vi "Main.vi"() -> ()   [LabVIEW 2020]
doc: "Application created to graph orbital movement of Venus, Earth, Mars and show distances and time needed for information to flow between them."
uses:
  Type Definitions/StateMachineEnum.ctl
  Variables/Stop-bool.vi
  Variables/Phi-initial.vi
panel:
  in  "Hiding button 2":bool
  in  "Hiding button":bool
  out "t S-E":string
  out "t M-E":string
  out "t S-M":string
  out "t V-M":string
  out "t S-V":string
  out "t V-E":string
  out "d M-E":dbl format="%.3g"
  out "d V-E":dbl format="%#.3g"
  out "d V-M":dbl format="%#.3g"
  out "d S-E":dbl format="%.3g"
  out "d S-M":dbl format="%.3g"
  out "d S-V":dbl format="%.3g"
  in  "Pause":bool
  out "Fi earth":dbl format="%#.4g"
  out "R earth":dbl format="%.4g"
  out "Fi mars":dbl format="%#.4g"
  out "R mars":dbl format="%.4g"
  out "Fi venus":dbl format="%#.4g"
  out "R venus":dbl format="%.4g"
  in  "Save Data":bool
  in  "Graphing speed":dbl(slide) scale=1.0..100.0
  out "XY Graph":cluster{dbl[], dbl[]}[](graph)
  in  "Stop drawing":bool
  in  "Draw Graph":bool
  in  "Exit":bool
  in  "Settings":bool
  # "Positions of planets"
  # "R [AU]"
  # "fi [deg]"
  # "Venus"
  # "Mars"
  # "Earth"
  # "Distances in AU (upper triangle) and time min::s::ms (lower triangle)"
  # "Sun"
  # "Venus"
  # "Mars"
  # "Earth"
  # "Sun"
  # "Venus"
  # "Mars"
  # "Earth"
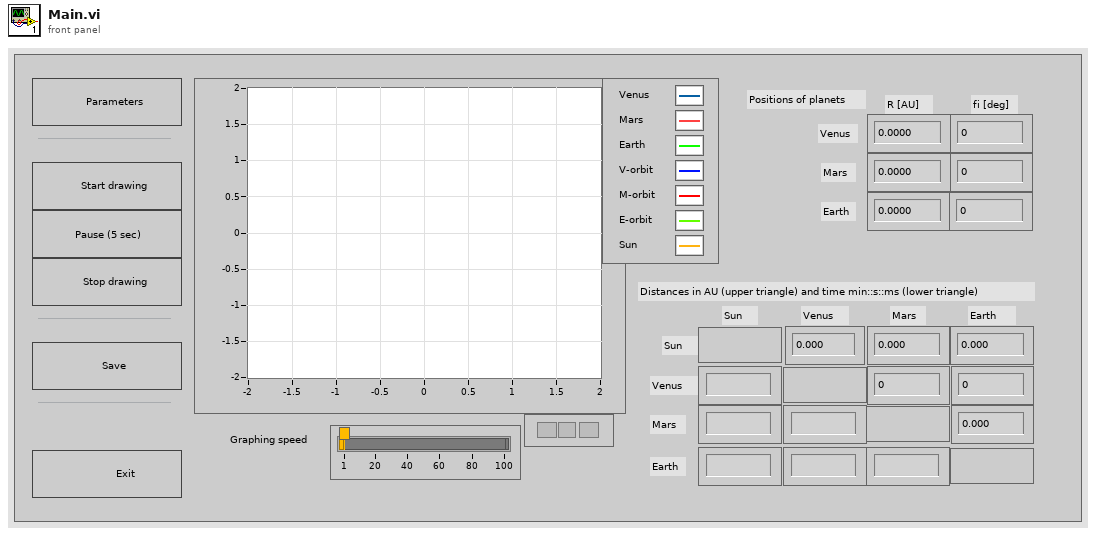
[diagram p1: front panel]
types:
  T1 = typedef "StateMachineEnum.ctl" = enum16{"Initialize", "Wait for event", "Draw graph", "Exit", "Save Data"}
  T2 = cluster{"t V-E":string, "t S-V":string, "t V-M":string, "t S-M":string, "t M-E":string, "t S-E":string}
  T3 = cluster{"d V-E":dbl, "d S-V":dbl, "d V-M":dbl, "d S-M":dbl, "d M-E":dbl, "d S-E":dbl}
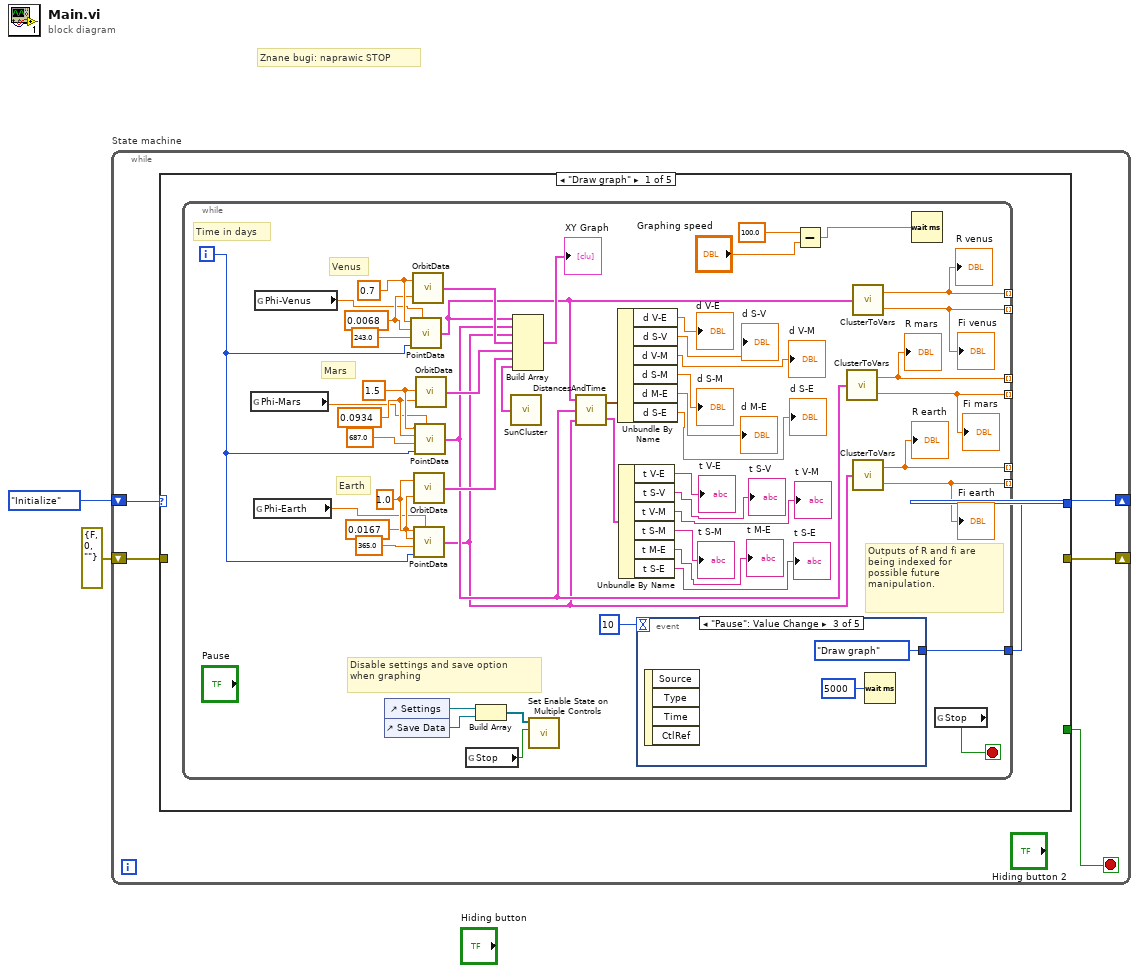
[diagram p0: block diagram]
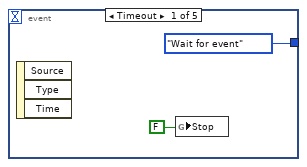
[diagram p2: hidden frame]
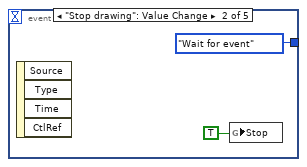
[diagram p3: hidden frame]
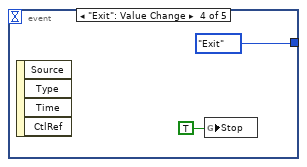
[diagram p4: hidden frame]
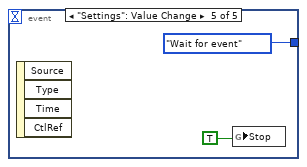
[diagram p5: hidden frame]
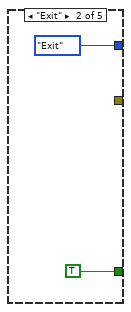
[diagram p6: hidden frame]
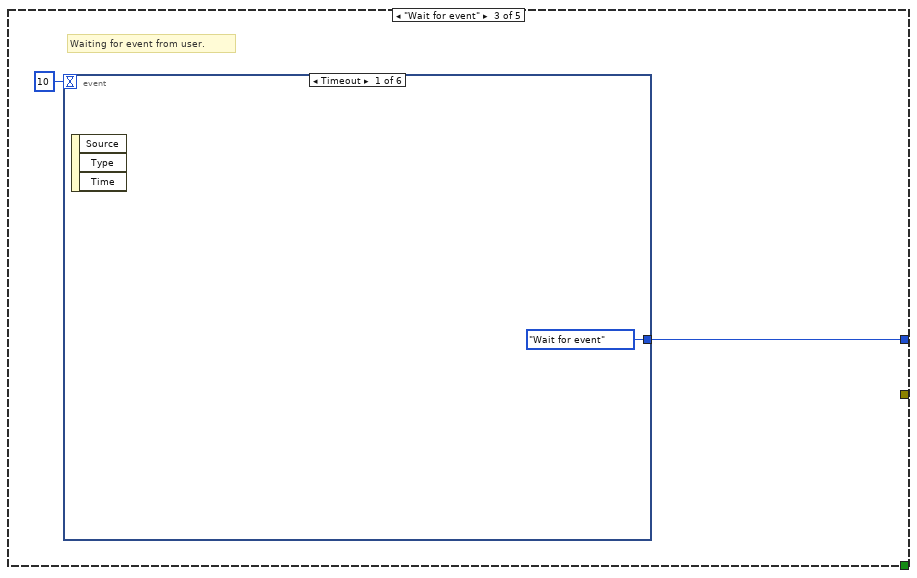
[diagram p7: hidden frame]
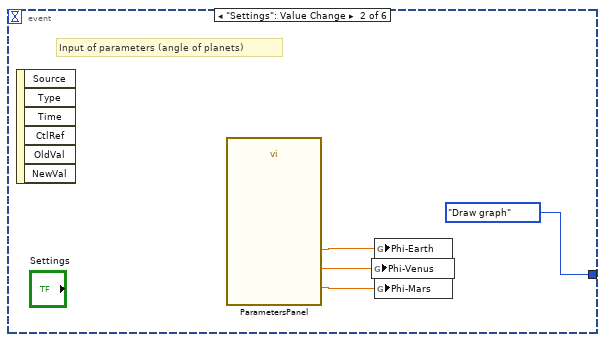
[diagram p8: hidden frame]
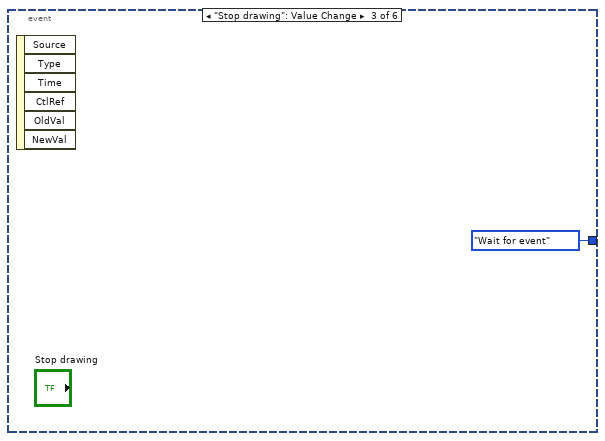
[diagram p9: hidden frame]
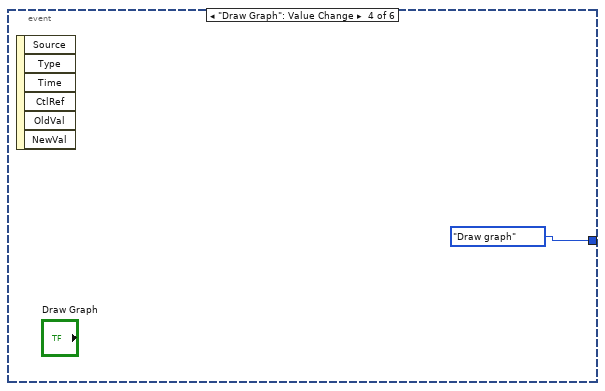
[diagram p10: hidden frame]
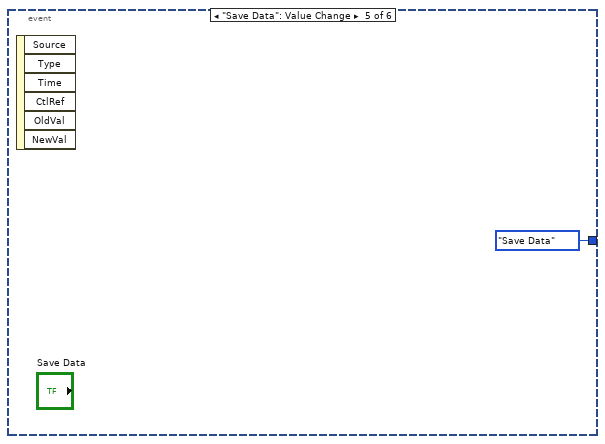
[diagram p11: hidden frame]
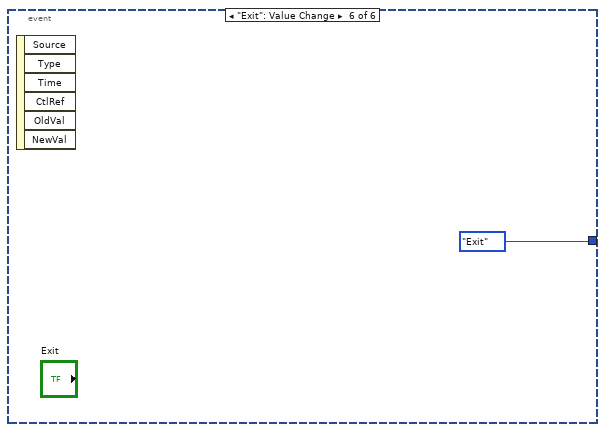
[diagram p12: hidden frame]
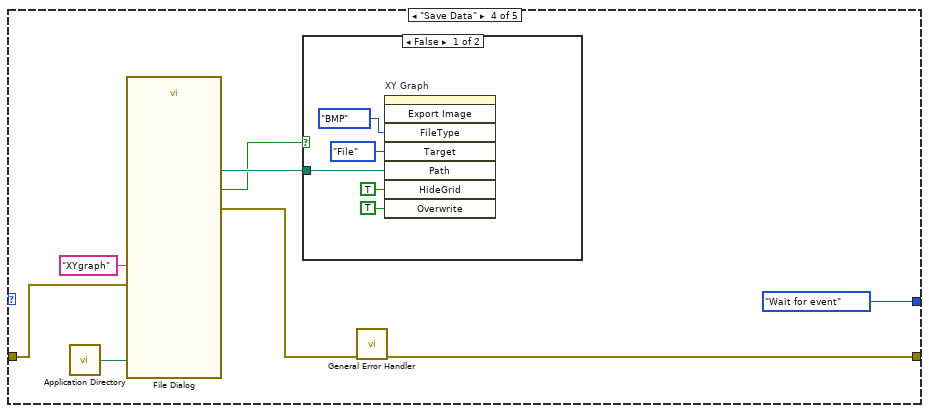
[diagram p13: hidden frame]
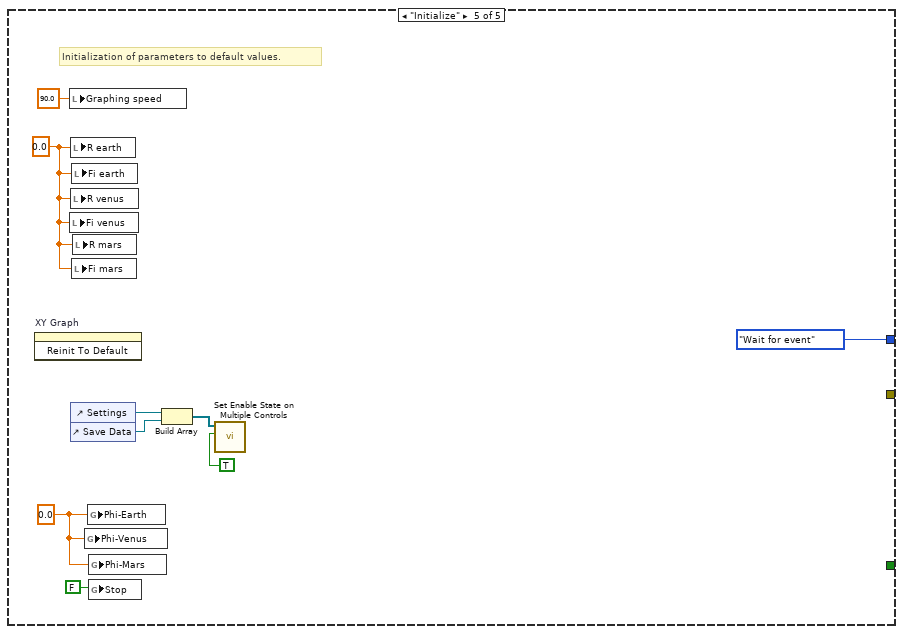
[diagram p15: hidden frame]
diagram:
  # "Znane bugi: naprawic STOP"
  n1 = while "State machine" {
    shift-right: [w5] -> _
    shift-left: StateMachineEnum."Initialize" -> [w7]
    shift-right: [w3] -> _
    shift-left: errorcluster {"status"=FALSE, "code"=0, "source"=""} ("error in") -> [w4]
    stop <- w6 stop-if-true
    n2 = case shown="\"Draw graph\"" w7 {
      tunnel: [w8 StateMachineEnum."Exit" w73 StateMachineEnum."Wait for event" StateMachineEnum."Wait for event"] -> w5
      tunnel: [_ TRUE _ _ _] -> w6
      tunnel: w4 -> [_ _ _ w85 _]
      tunnel: [_ _ _ w83 _] -> w3
      frame "Draw graph" {
        n3 = while {
          tunnel: [w59] -> w8
          tunnel: [w27] -> _ mode=indexing
          tunnel: [w26] -> _ mode=indexing
          tunnel: [w29] -> _ mode=indexing
          tunnel: [w28] -> _ mode=indexing
          tunnel: [w31] -> _ mode=indexing
          tunnel: [w30] -> _ mode=indexing
          i -> [w40]
          stop <- w57 stop-if-true
          w46 = 0.7 ("a")
          w47 = 1.5 ("a")
          w49 = 1.0 ("a")
          w44 = 0.0934 ("e")
          w45 = 0.0068 ("e")
          w48 = 0.0167 ("e")
          # "Outputs of R and fi are\nbeing indexed for \npossible future \nmanipulation."
          # "Disable settings and save option\nwhen graphing"
          # "Time in days"
          # "Venus"
          # "Mars"
          # "Earth"
          n4 = global read "Phi-initial.vi" "Phi-Mars"() -> (w38:dbl)
          n5 = global read "Phi-initial.vi" "Phi-Earth"() -> (w37:dbl)
          n6 = global read "Phi-initial.vi" "Phi-Venus"() -> (w39:dbl)
          n7 = control-ref of="Settings"() -> (w35:refnum<vi>)
          n8 = control-ref of="Save Data"() -> (w33:refnum<vi>)
          n9 = call "PointData.vi"("a"=w46, "e"=w45, "Period"=243.0, "time in days"=w40, "Initial fi"=w39) -> ("Cluster XY"=w25:cluster{dbl[], dbl[]})
          n10 = call "OrbitData.vi"("e"=w45, "a"=w46) -> ("Orbit XY"=w52:cluster{dbl[], dbl[]})
          n11 = call "OrbitData.vi"("e"=w48, "a"=w49) -> ("Orbit XY"=w50:cluster{dbl[], dbl[]})
          n12 = call "PointData.vi"("a"=w49, "e"=w48, "Period"=365.0, "time in days"=w40, "Initial fi"=w37) -> ("Cluster XY"=w23:cluster{dbl[], dbl[]})
          n13 = call "PointData.vi"("a"=w47, "e"=w44, "Period"=687.0, "time in days"=w40, "Initial fi"=w38) -> ("Cluster XY"=w24:cluster{dbl[], dbl[]})
          n14 = call "OrbitData.vi"("e"=w44, "a"=w47) -> ("Orbit XY"=w51:cluster{dbl[], dbl[]})
          n15 = global read "Stop-bool.vi" "Stop"() -> (w34:bool)
          n16 = Build Array(w35, w33) -> (w36:refnum<vi>[])
          n17 = call "SunCluster.vi"() -> ("XY Sun Cluster"=w32:cluster{dbl[], dbl[]})
          n18 = Build Array(w25, w24, w23, w52, w51, w50, w32) -> (→"XY Graph":cluster{dbl[], dbl[]}[])
          n19 = call "Set Enable State on Multiple Controls.vi"("Enable?"=w34, "Controls"=w36) -> ()  [unwired: 10 in]
          n20 = call "DistancesAndTime.vi"("Cluster XY Earth"=w23, "Cluster XY Mars"=w24, "Cluster XY Venus"=w25) -> ("time cluster"=w15:T2, "distance cluster"=w22:T3)
          n21 = Unbundle By Name(w22) -> ("d V-E"=→"d V-E":dbl, "d S-V"=→"d S-V":dbl, "d V-M"=→"d V-M":dbl, "d S-M"=→"d S-M":dbl, "d M-E"=→"d M-E":dbl, "d S-E"=→"d S-E":dbl)
          n22 = Unbundle By Name(w15) -> ("t V-E"=→"t V-E":string, "t S-V"=→"t S-V":string, "t V-M"=→"t V-M":string, "t S-M"=→"t S-M":string, "t M-E"=→"t M-E":string, "t S-E"=→"t S-E":string)
          n23 = event shown="[2] \"Pause\": Value Change" {
            selector: _ -> [_ _ _ _ _]
            dyn-events: _ -> [_ _ _ _ _]
            timeout: 10 -> [_ _ _ _ _]
            tunnel: [StateMachineEnum."Wait for event" StateMachineEnum."Wait for event" StateMachineEnum."Draw graph" StateMachineEnum."Exit" StateMachineEnum."Wait for event"] -> w59
            event Timeout {
              n24 = event-data() -> ()  [unwired: 1 in, 3 out]
              n25 = global write "Stop-bool.vi" "Stop"(FALSE) -> ()
            }
            event "Stop drawing": Value Change {
              n26 = event-data() -> ()  [unwired: 1 in, 4 out]
              n27 = global write "Stop-bool.vi" "Stop"(TRUE) -> ()
            }
            event "Pause": Value Change {
              n28 = event-data() -> ()  [unwired: 1 in, 4 out]
              n29 = Wait (ms)(milliseconds to wait=u32 5000) -> ()  [unwired: 1 out]
            }
            event "Exit": Value Change {
              n30 = event-data() -> ()  [unwired: 1 in, 4 out]
              n31 = global write "Stop-bool.vi" "Stop"(TRUE) -> ()
            }
            event "Settings": Value Change {
              n32 = event-data() -> ()  [unwired: 1 in, 4 out]
              n33 = global write "Stop-bool.vi" "Stop"(TRUE) -> ()
            }
          }
          n34 = Subtract(x=100.0, y="Graphing speed") -> (x-y=w53:dbl)
          n35 = call "ClusterToVars.vi"("Cluster XY"=w24) -> ("R value"=w29:dbl, "Fi value"=w28:dbl)
          "R mars" <- w29
          "Fi mars" <- w28
          n36 = call "ClusterToVars.vi"("Cluster XY"=w25) -> ("R value"=w27:dbl, "Fi value"=w26:dbl)
          "R venus" <- w27
          "Fi venus" <- w26
          n37 = call "ClusterToVars.vi"("Cluster XY"=w23) -> ("R value"=w31:dbl, "Fi value"=w30:dbl)
          "R earth" <- w31
          "Fi earth" <- w30
          n38 = Wait (ms)(milliseconds to wait=w53) -> ()  [unwired: 1 out]
          n39 = global read "Stop-bool.vi" "Stop"() -> (w57:bool)
        }
      }
      frame "Exit" {
      }
      frame "Wait for event" {
        # "Waiting for event from user."
        n40 = event shown="[0] Timeout" {
          selector: _ -> [_ _ _ _ _ _]
          dyn-events: _ -> [_ _ _ _ _ _]
          timeout: 10 -> [_ _ _ _ _ _]
          tunnel: [StateMachineEnum."Wait for event" StateMachineEnum."Draw graph" StateMachineEnum."Wait for event" StateMachineEnum."Draw graph" StateMachineEnum."Save Data" StateMachineEnum."Exit"] -> w73
          event Timeout {
            n41 = event-data() -> ()  [unwired: 1 in, 3 out]
          }
          event "Settings": Value Change {
            # "Input of parameters (angle of planets)"
            n42 = event-data() -> ()  [unwired: 1 in, 6 out]
            n43 = call "ParametersPanel.vi"() -> ("fi - Mars"=w76:dbl, "fi - Venus"=w77:dbl, "fi - Earth"=w78:dbl)  [unwired: 15 in, 2 out]
            n44 = global write "Phi-initial.vi" "Phi-Venus"(w77) -> ()
            n45 = global write "Phi-initial.vi" "Phi-Earth"(w78) -> ()
            n46 = global write "Phi-initial.vi" "Phi-Mars"(w76) -> ()
          }
          event "Stop drawing": Value Change {
            n47 = event-data() -> ()  [unwired: 1 in, 6 out]
          }
          event "Draw Graph": Value Change {
            n48 = event-data() -> ()  [unwired: 1 in, 6 out]
          }
          event "Save Data": Value Change {
            n49 = event-data() -> ()  [unwired: 1 in, 6 out]
          }
          event "Exit": Value Change {
            n50 = event-data() -> ()  [unwired: 1 in, 6 out]
          }
        }
      }
      frame "Save Data" {
        n51 = call <vilib>:"Application Directory.vi"() -> ("Application Directory"=w86:path)
        n52 = call "File Dialog"("start path"=w86, "default name"="XYgraph", "error in"=w85) -> ("selected path"=w89:path, "cancelled"=w88:bool, "error out"=w84:errorcluster)  [unwired: 9 in, 1 out]
        n53 = case shown="False" w88 {
          tunnel: w89 -> [w91 _]
          frame False {
            n54 = invoke on="XY Graph" class="XYGraph (strict)" method="Export Image"("FileType"=enum32{"BMP", "EPS", "EMF", "PICT"}."BMP" ("File Type"), "Target"=enum32{"File", "Clipboard"}."File", "Path"=w91, "HideGrid"=TRUE ("Hide Grid"), "Overwrite"=TRUE ("Always Overwrite")) -> ()  [unwired: 3 in, 8 out]
          }
          frame True {
          }
        }
        n55 = call <vilib>:"General Error Handler.vi"("error in (no error)"=w84) -> ("error out"=w83:errorcluster)  [unwired: 10 in, 4 out]
      }
      frame "Initialize" {
        w98 = 0.0 ("X earth")
        w96 = 0.0 ("Phi-Earth")
        # "Initialization of parameters to default values."
        n56 = invoke on="XY Graph" class="XYGraph (strict)" method="Reinit To Default"() -> ()  [unwired: 3 in, 3 out]
        n57 = local write "Graphing speed"(90.0 ("Graphing speed")) -> ()
        n58 = local write "Fi venus"(w98) -> ()
        n59 = local write "R earth"(w98) -> ()
        n60 = local write "R venus"(w98) -> ()
        n61 = control-ref of="Settings"() -> (w100:refnum<vi>)
        n62 = control-ref of="Save Data"() -> (w102:refnum<vi>)
        n63 = local write "Fi earth"(w98) -> ()
        n64 = local write "Fi mars"(w98) -> ()
        n65 = local write "R mars"(w98) -> ()
        n66 = global write "Phi-initial.vi" "Phi-Venus"(w96) -> ()
        n67 = global write "Phi-initial.vi" "Phi-Earth"(w96) -> ()
        n68 = global write "Phi-initial.vi" "Phi-Mars"(w96) -> ()
        n69 = global write "Stop-bool.vi" "Stop"(FALSE ("Stop")) -> ()
        n70 = Build Array(w100, w102) -> (w101:refnum<vi>[])
        n71 = call "Set Enable State on Multiple Controls.vi"("Enable?"=TRUE, "Controls"=w101) -> ()  [unwired: 10 in]
      }
    }
  }
